vi "Stop Core.vi"(10 "final error code":i32, 11 "Reference Range Actor in":refnum<class "Reference Range Actor.lvclass">) -> (3 "Reference Range Actor out":refnum<class "Reference Range Actor.lvclass">)   [LabVIEW 2018, in "Reference Range.lvlib" / "Reference Range Actor.lvclass"]
doc: "(<B>Filename</B>: Actor Framework.lvlib:Actor.lvclass:Stop Core.vi)\n\nDefines what the actor does before it stops. Use the <B>final error code</B> input to determine whether the actor shut down in response to an error.\n\nBy default, this method does nothing. A descendant class may override it to define behavior, such as shutting down any processes the actor initiated in its override of the Actor Core method."
uses:
  Reference Range Actor.lvclass
  Reference Range Actor.lvclass/Reference Range Actor.ctl
  Actor Monitor/Actor/Monitored Actor.lvclass
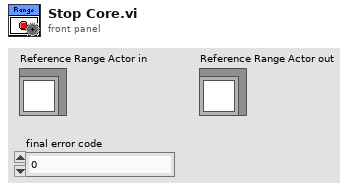
[diagram p1: front panel]
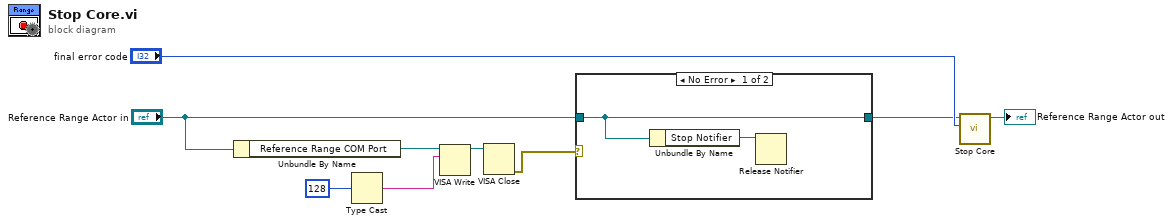
[diagram p0: block diagram]
diagram:
  n1 = Unbundle By Name("Reference Range Actor in") -> ("Reference Range COM Port"=w8:refnum<visa-resource-name>)
  n2 = Type Cast(x=i16 128) -> (*(type *) &x=w6:string)  [unwired: 1 in]
  n3 = VISA Write(VISA resource name=w8, write buffer=w6) -> (VISA resource name out=w7:refnum<visa-resource-name>)  [unwired: 1 in, 2 out]
  n4 = VISA Close(VISA resource name=w7) -> (error out=w1:errorcluster)  [unwired: 1 in]
  n5 = case shown="No Error" w1 {
    tunnel: "Reference Range Actor in" -> [w11 w12]
    tunnel: [w11 w12] -> w2
    frame No Error {
      n6 = Unbundle By Name(w11) -> ("Stop Notifier"=w10:refnum<notifier>)
      n7 = Release Notifier(notifier=w10) -> ()  [unwired: 2 in, 3 out]
    }
    frame Error {
    }
  }
  n8 = call-parent "Stop Core.vi"("final error code"="final error code", "Monitored Actor in"=w2) -> ("Monitored Actor out"=→"Reference Range Actor out":refnum<class "Reference Range Actor.lvclass">)  [unwired: 9 in]
